vi "test harness_FXP_L_ye_Bend_u_singleAxis_REAL_DATA.vi"(8 "error in (no error)":errorcluster, 11 "TestCase in":refnum<class "FXP_observer_TestCase.lvclass">) -> (0 "error out":errorcluster, 3 "TestCase out":refnum<class "FXP_observer_TestCase.lvclass">)   [LabVIEW 2017, in "FXP_observer_TestCase.lvclass"]
uses:
  FXP_observer_TestCase.lvclass
  <vilib>/rvi/DesktopExecutionNode/Execution/niFpgaDEN_Execute.vi
  <vilib>/rvi/DesktopExecutionNode/DesktopExecutionNode.xnode
  <vilib>/addons/_JKI Toolkits/VI Tester/TestCase.llb/TestCase.lvclass
  C:/Program Files (x86)/National Instruments/LabVIEW 2017/vi.lib/addons/_JKI Toolkits/VI Tester/TestCase.llb/TestCase.lvclass
panel:
  out "x+y":fxp<+/-,51,11>[](array[numeric])
  out "xk_1_1":fxp<+/-,32,5>[](array[numeric])
  out "error (x_1_1)":errorcluster
  out "error (xu)":errorcluster
  out "error (yd)":errorcluster
  in  "x_u(k)":fxp<+/-,32,8>=13.600000023841858
  in  "U(k): ux":fxp<+/-,18,5>=0.14501953125
  in  "y(k)":fxp<+/-,18,5>=0.123046875
  in  "NS":u8=5
  # "Remember that Ldist and Bz only have\ntwo integer bits!"
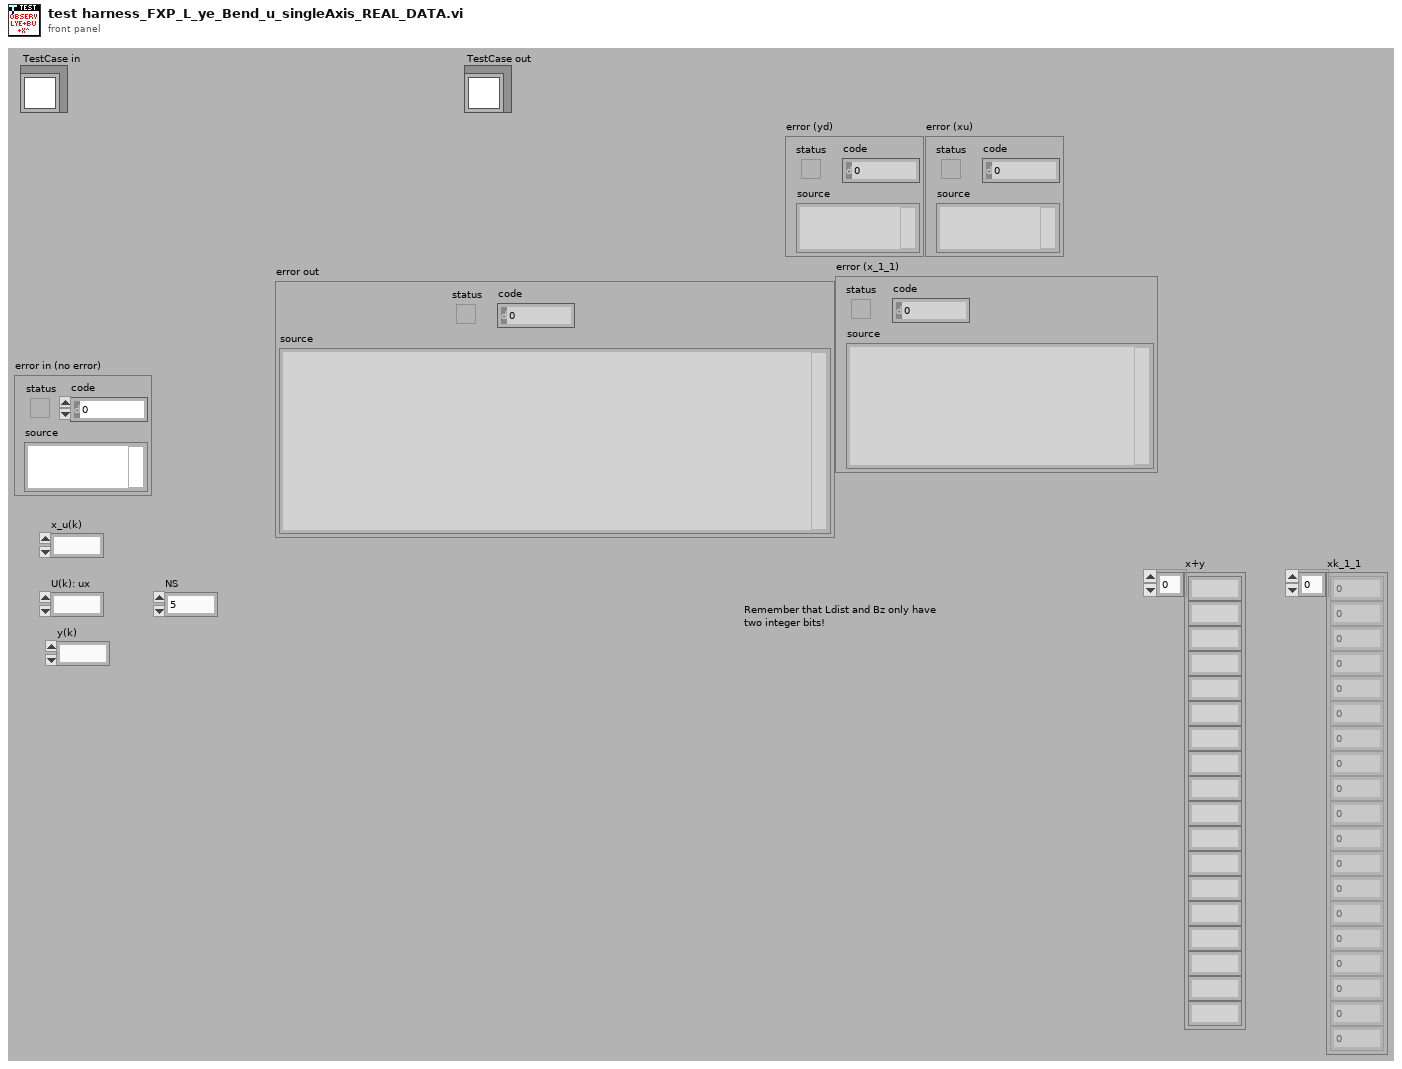
[diagram p1: front panel]
types:
  T1 = typedef "UT_matrix_data.ctl" = cluster{"Bz":T2[], "Ldist":T3[], "Kz":T4[], "Nx":T5[], "Ax_col":T6[], "X_vec":T7[], "Cz":T8[]}
  T2 = typedef "Bz_vec_scalar.ctl" = fxp<+/-,32,3>
  T3 = typedef "Lz_vec_scalar.ctl" = fxp<+/-,32,3>
  T4 = typedef "Kz_vec_scalar.ctl" = fxp<+/-,32,10>
  T5 = typedef "Nx_vec_scalar.ctl" = fxp<+/-,32,2>
  T6 = typedef "Az_vec_scalar.ctl" = fxp<+/-,32,7>
  T7 = typedef "x_vec_scalar.ctl" = fxp<+/-,32,6>
  T8 = typedef "Cz_vec_scalar.ctl" = fxp<+/-,32,4>
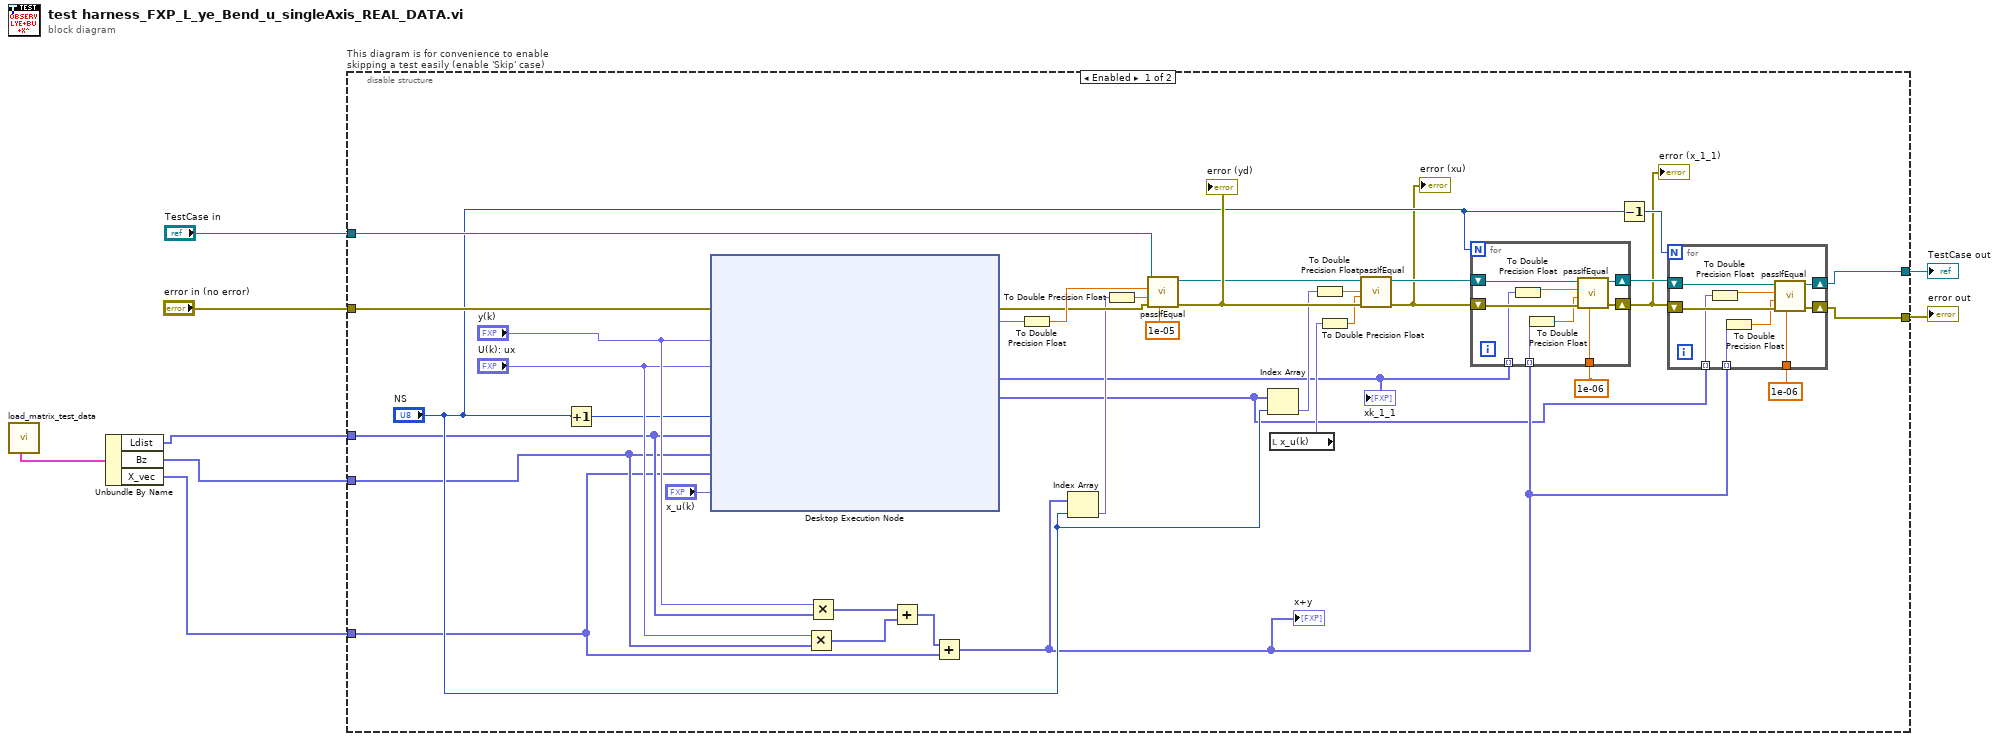
[diagram p0: block diagram]
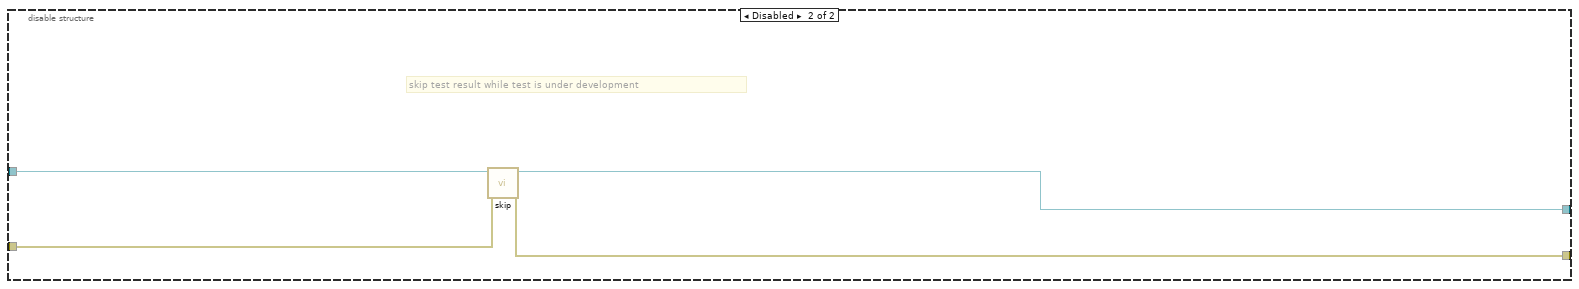
[diagram p2: hidden frame]
diagram:
  n1 = call "load_matrix_test_data.vi"() -> ("output cluster"=w4:T1)  [unwired: 5 in, 6 out]
  n2 = Unbundle By Name(w4) -> ("Ldist"=w3:T3[], "Bz"=w2:T2[], "X_vec"=w1:T7[])
  n3 = disable-structure "This diagram is for convenience to enable skipping a test easily (enable 'Skip' case)" shown="Enabled" {
    disable-tunnel: "TestCase in" -> [w45 w67]
    disable-tunnel: [w20 w65] -> w5
    disable-tunnel: [w19 w66] -> w7
    disable-tunnel: "error in (no error)" -> [w41 w64]
    disable-tunnel: w3 -> [w11 _]
    disable-tunnel: w2 -> [w10 _]
    disable-tunnel: w1 -> [w9 _]
    frame Enabled {
      n4 = Increment(x="NS") -> (x+1=w32:u8)
      n5 = xnode "Desktop Execution Node"("Error In"=w41, "y(k)"="y(k)", "U(k): ux"="U(k): ux", "NS + 1"=w32, "Ldist"=w11, "Bz"=w10, "x"=w9, "x_u(k)"="x_u(k)") -> ("Error Out"=w42:errorcluster, "yd_est"=w35:fxp<+/-,32,5>, "xk_1_1"=w23:fxp<+/-,32,5>[], "xk_1_2"=w14:fxp<+/-,32,5>[])
      "xk_1_1" <- w23
      n6 = Multiply(x="U(k): ux", y=w10) -> (x*y=w37:fxp<+/-,50,8>[])
      n7 = Multiply(x="y(k)", y=w11) -> (x*y=w38:fxp<+/-,50,8>[])
      n8 = Add(x=w38, y=w37) -> (x+y=w36:fxp<+/-,51,9>[])
      n9 = Add(x=w36, y=w9) -> (x+y=w15:fxp<+/-,51,9>[])
      "x+y" <- w15
      n10 = To Double Precision Float(number=w35) -> (double precision float=w43:dbl)
      n11 = Index Array(array=w15, index="NS") -> (element=w33:fxp<+/-,51,9>)
      n12 = To Double Precision Float(number=w33) -> (double precision float=w34:dbl)
      n13 = call-dynamic "passIfEqual.vi"("delta (optional)"=1e-05 ("del u_x"), "error in (no error)"=w42, "y"=w34, "x"=w43, "TestCase in"=w45) -> ("error out"=w30:errorcluster, "TestCase out"=w29:refnum<class "FXP_observer_TestCase.lvclass">)  [unwired: 5 in]
      "error (yd)" <- w30
      n14 = Index Array(array=w14, index="NS") -> (element=w27:fxp<+/-,32,5>)
      n15 = local read "x_u(k)"() -> (w25:fxp<+/-,32,8>)
      n16 = To Double Precision Float(number=w27) -> (double precision float=w28:dbl)
      n17 = To Double Precision Float(number=w25) -> (double precision float=w26:dbl)
      n18 = call-dynamic "passIfEqual.vi"("error in (no error)"=w30, "y"=w26, "x"=w28, "TestCase in"=w29) -> ("error out"=w13:errorcluster, "TestCase out"=w24:refnum<class "FXP_observer_TestCase.lvclass">)  [unwired: 6 in]
      "error (xu)" <- w13
      n19 = for {
        N: "NS" -> [_]
        shift-right: [w63] -> w21
        shift-left: w24 -> [w60]
        shift-right: [w62] -> w12
        shift-left: w13 -> [w61]
        tunnel: w15 -> [w59] mode=indexing
        tunnel: w23 -> [w56] mode=indexing
        tunnel: 1e-06 ("del u_x") -> [w55]
        n20 = To Double Precision Float(number=w56) -> (double precision float=w57:dbl)
        n21 = To Double Precision Float(number=w59) -> (double precision float=w58:dbl)
        n22 = call-dynamic "passIfEqual.vi"("delta (optional)"=w55, "error in (no error)"=w61, "y"=w58, "x"=w57, "TestCase in"=w60) -> ("error out"=w62:errorcluster, "TestCase out"=w63:refnum<class "FXP_observer_TestCase.lvclass">)  [unwired: 5 in]
      }
      "error (x_1_1)" <- w12
      n23 = Decrement(x="NS") -> (x-1=w17:u8)
      n24 = for {
        N: w17 -> [_]
        shift-right: [w54] -> w20
        shift-left: w21 -> [w51]
        shift-right: [w53] -> w19
        shift-left: w12 -> [w52]
        tunnel: w15 -> [w50] mode=indexing
        tunnel: w14 -> [w47] mode=indexing
        tunnel: 1e-06 ("del u_x") -> [w46]
        n25 = To Double Precision Float(number=w47) -> (double precision float=w48:dbl)
        n26 = To Double Precision Float(number=w50) -> (double precision float=w49:dbl)
        n27 = call-dynamic "passIfEqual.vi"("delta (optional)"=w46, "error in (no error)"=w52, "y"=w49, "x"=w48, "TestCase in"=w51) -> ("error out"=w53:errorcluster, "TestCase out"=w54:refnum<class "FXP_observer_TestCase.lvclass">)  [unwired: 5 in]
      }
    }
    frame Disabled {
      # "skip test result while test is under development"
      n28 = call <vilib>:"skip.vi"("error in (no error)"=w64, "TestCase in"=w67) -> ("error out"=w66:errorcluster, "TestCase out"=w65:refnum<class "FXP_observer_TestCase.lvclass">)  [unwired: 8 in]
    }
  }
  "error out" <- w7
  "TestCase out" <- w5
